vi "Close Front Panel.vi"(8 "error in (no error)":errorcluster, 10 "Hide? (F)":bool, 11 "IViewable in":refnum<class "IViewable.lvclass">) -> (0 "error out":errorcluster, 3 "IViewable out":refnum<class "IViewable.lvclass">)   [LabVIEW 2017, in "IViewable.lvlib" / "IViewable.lvclass"]
doc: "<License>\nCopyright © 2017 Composed Systems, LLC | All rights reserved\nwww.composed.io\n\nAuthor: Ethan Stern <ethan.stern@composed.io>\n\nThis software is provided \"AS IS\" WITHOUT WARRANTIES, either express or implied, AND IS FOR EDUCATIONAL PURPOSES ONLY.\n</License>"
uses:
  IViewable.lvclass
  IViewable.lvclass/IViewable.ctl
  ProtectedSubpanel/Protected Subpanel Reference.ctl
  ProtectedSubpanel/ProtectedSubpanel.lvclass
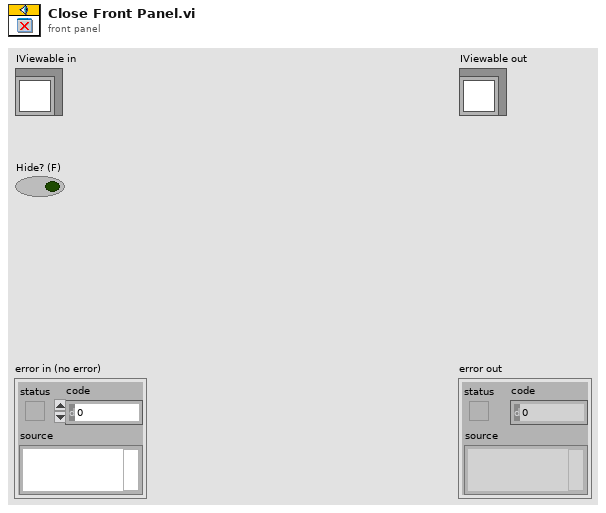
[diagram p1: front panel]
types:
  T1 = typedef "IViewable.lvlib/ProtectedSubpanel.lvclass/Protected Subpanel Reference.ctl" = refnum<data-value>
  T2 = enum32{"Invalid", "Standard", "Closed", "Hidden", "Minimized", "Maximized"}
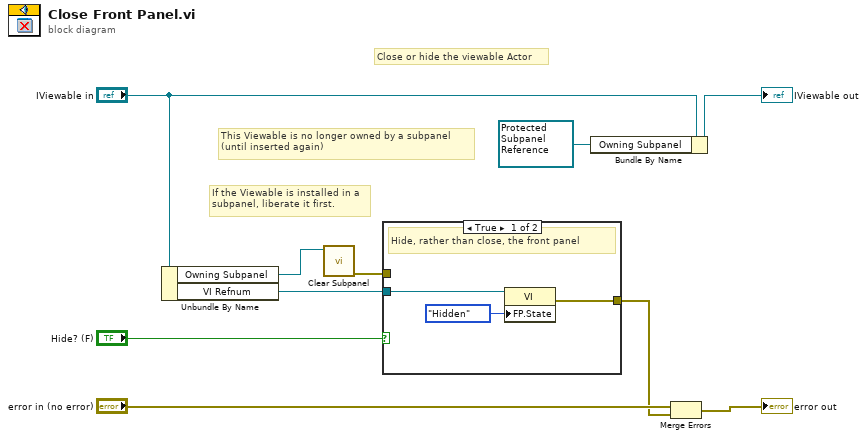
[diagram p0: block diagram]
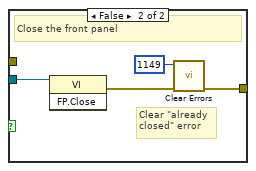
[diagram p2: hidden frame]
diagram:
  # "This Viewable is no longer owned by a subpanel\n(until inserted again)"
  # "If the Viewable is installed in a\nsubpanel, liberate it first."
  # "Close or hide the viewable Actor"
  n1 = Unbundle By Name("IViewable in") -> ("Owning Subpanel"=w4:T1, "VI Refnum"=w6:refnum<vi>)
  n2 = call "Clear Subpanel.vi"("Protected Subpanel"=w4) -> ("error out"=w3:errorcluster)  [unwired: 9 in, 1 out]
  n3 = case shown="True" "Hide? (F)" {
    tunnel: [w13 w15] -> w7
    tunnel: w6 -> [w12 w16]
    tunnel: w3 -> [_ _]
    frame True {
      # "Hide, rather than close, the front panel"
      n4 = property class="VI"(reference=w12, "FP.State"=T2."Hidden" ("Front Panel Window:State")) -> (error out=w13:errorcluster)  [unwired: 1 in, 1 out]
    }
    frame False {
      # "Clear \"already \nclosed\" error"
      # "Close the front panel"
      n5 = invoke class="VI" method="FP.Close"(reference=w16) -> (error out=w17:errorcluster)  [unwired: 2 in, 2 out]
      n6 = call <vilib>:"Clear Errors.vi"("error in (no error)"=w17, "specific error code to clear (0: all)"=1149) -> ("error out"=w15:errorcluster)  [unwired: 4 in, 1 out]
    }
  }
  n7 = Bundle By Name(cluster="IViewable in", "Owning Subpanel"=T1 refnum) -> (→"IViewable out":refnum<class "IViewable.lvclass">)
  n8 = Merge Errors("error in (no error)", w7) -> (→"error out":errorcluster)
